vi "generated_from_signal_express.vi"() -> (3 "Voltage":waveform(dbl)[](array[waveform]) caption="data out")   [LabVIEW 2013]
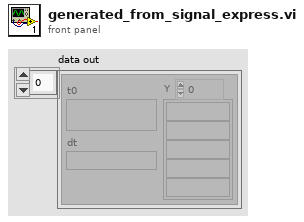
[diagram p1: front panel]
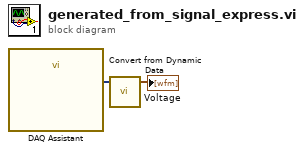
[diagram p0: block diagram]
diagram:
  n1 = call "DAQ Assistant"() -> ("data"=w2:dynamicdata)  [unwired: 16 in, 3 out]
  n2 = call "Convert from Dynamic Data"("Dynamic Data Type"=w2) -> ("Array of Waveform"=→"Voltage":waveform(dbl)[])  [unwired: 3 in]
